vi "GOOP_CurrentProviderClass_ReadDefault.vi"(0 "GetThisClassProvidersPaths(Returns the default providor if not wired)":string, 11 "error in":errorcluster) -> (4 "value":string, 6 "Writer":path, 8 "Reader":path, 14 "Providers":string[](array[string]), 15 "error out":errorcluster)   [LabVIEW 2020]
uses:
  <vilib>/Utility/config.llb/Read Key (String).vi
  <vilib>/Utility/config.llb/NI_LVConfig.lvlib
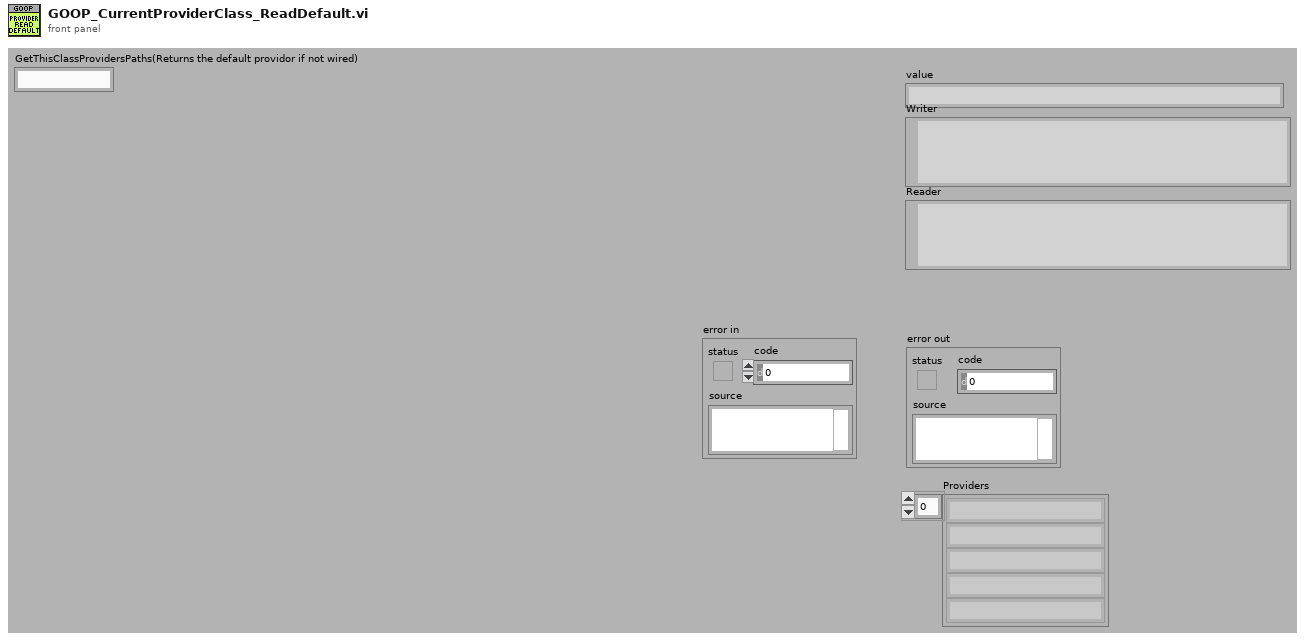
[diagram p1: front panel]
types:
  T1 = typedef "NI_LVConfig.lvlib/Config Data RefNum.ctl" = refnum<k1>
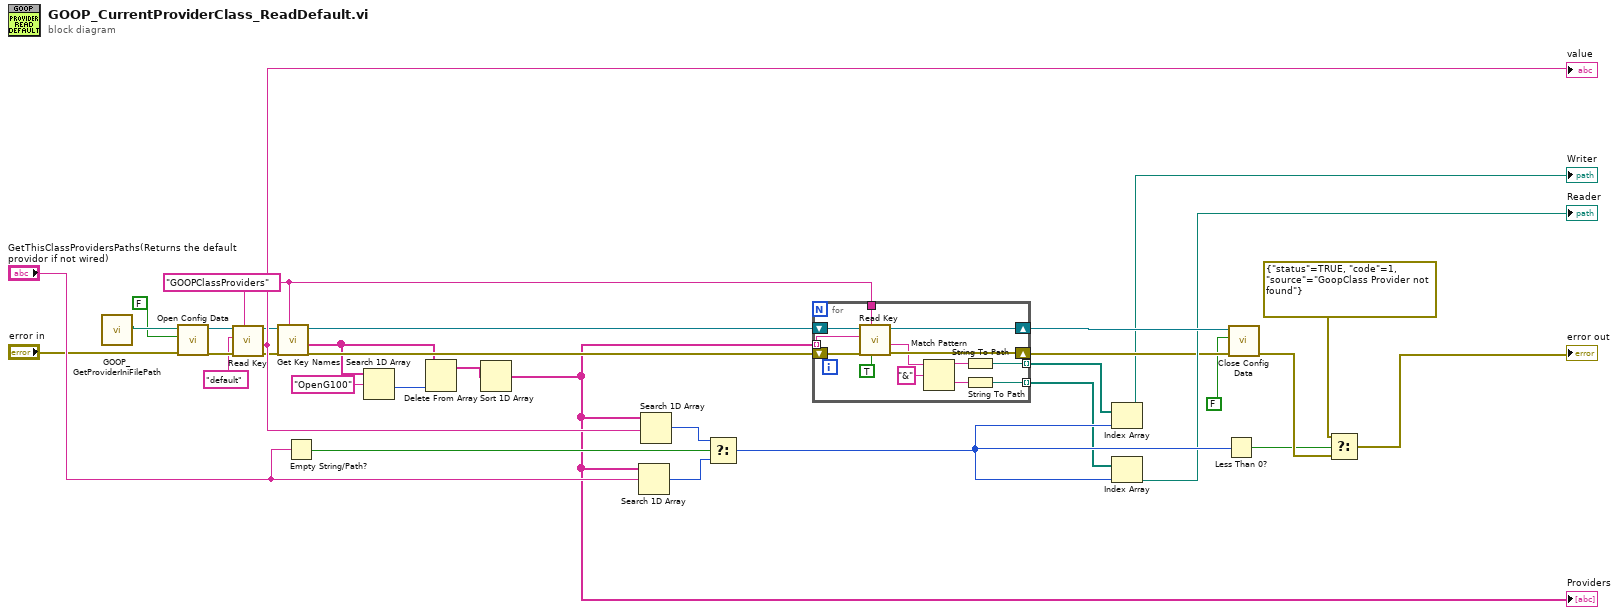
[diagram p0: block diagram]
diagram:
  w18 = "GOOPClassProviders" ("section")
  n1 = call <resource>:"GOOP_GetProviderIniFilePath.vi"() -> ("ProviderIniPath"=w12:path)  [unwired: 10 in, 1 out]
  n2 = call <vilib>:"Open Config Data.vi"("error in (no error)"="error in", "create file if necessary (T)"=FALSE ("create file if necessary? (T)"), "configuration file path"=w12) -> ("error out"=w9:errorcluster, "refnum"=w7:T1)  [unwired: 6 in, 1 out]
  n3 = call-poly <vilib>:"Read Key.vi"("section"=w18, "error in (no error)"=w9, "key"="default", "refnum"=w7) -> ("error out"=w14:errorcluster, "value"=w24:string, "refnum out"=w13:T1)  [unwired: 4 in, 1 out]
  "value" <- w24
  n4 = call <vilib>:"Get Key Names.vi"("section"=w18, "error in (no error)"=w14, "refnum"=w13) -> ("error out"=w16:errorcluster, "key names"=w4:string[], "refnum out"=w17:T1)  [unwired: 5 in, 1 out]
  n5 = Empty String/Path?(string/path="GetThisClassProvidersPaths(Returns the default providor if not wired)") -> (empty?=w30:bool)
  n6 = Search 1D Array(1D array=w4, element="OpenG100") -> (index of element=w3:i32)  [unwired: 1 in]
  n7 = Delete From Array(array=w4, index=w3) -> (array with subset deleted=w2:string[])  [unwired: 1 in, 1 out]
  n8 = Sort 1D Array(array=w2) -> (sorted array=w1:string[])
  "Providers" <- w1
  n9 = Search 1D Array(1D array=w1, element="GetThisClassProvidersPaths(Returns the default providor if not wired)") -> (index of element=w32:i32)  [unwired: 1 in]
  n10 = Search 1D Array(1D array=w1, element=w24) -> (index of element=w31:i32)  [unwired: 1 in]
  n11 = Select(t=w31, s=w30, f=w32) -> (s? t:f=w33:i32)
  n12 = for {
    tunnel: w1 -> [w46] mode=indexing
    shift-right: [w44] -> w20
    shift-left: w16 -> [w45]
    shift-right: [w42] -> w23
    shift-left: w17 -> [w43]
    tunnel: w18 -> [w41]
    tunnel: [w36] -> w19 mode=indexing
    tunnel: [w34] -> w21 mode=indexing
    n13 = call-poly <vilib>:"Read Key.vi"("read raw string? (F)"=TRUE, "section"=w41, "error in (no error)"=w45, "key"=w46, "refnum"=w43) -> ("error out"=w44:errorcluster, "value"=w39:string, "refnum out"=w42:T1)  [unwired: 3 in, 1 out]
    n14 = Match Pattern(string=w39, regular expression="&") -> (before substring=w37:string, after substring=w35:string)  [unwired: 1 in, 2 out]
    n15 = String To Path(string=w37) -> (path=w36:path)
    n16 = String To Path(string=w35) -> (path=w34:path)
  }
  n17 = Index Array(array=w19, index=w33) -> (element=→"Writer":path)
  n18 = Index Array(array=w21, index=w33) -> (element=→"Reader":path)
  n19 = Less Than 0?(x=w33) -> (x < 0?=w25:bool)
  n20 = call <vilib>:"Close Config Data.vi"("error in (no error)"=w20, "write file if changed (T)"=FALSE ("write configuration file? (T)"), "refnum"=w23) -> ("error out"=w26:errorcluster)  [unwired: 7 in, 1 out]
  n21 = Select(t=errorcluster {"status"=TRUE, "code"=1, "source"="GoopClass Provider not found"}, s=w25, f=w26) -> (s? t:f=→"error out":errorcluster)
